vi "add data indicies controls.vi"(8 "error in":errorcluster, 9 "Channels to create":T1[](array[typedef]), 10 "runtime class path":path, 11 "Application in":refnum<vi>) -> (0 "error out":errorcluster)   [LabVIEW 2013, in "FixedChannelTBModuleDecideFeatures.lvclass"]
uses:
  FixedChannelTBModuleDecideFeatures.lvclass
  <vilib>/NI/Tag Bus Module Framework/channel/channel classification.ctl
  <vilib>/NI/Tag Bus Module Framework/channel/TBM channel.lvclass
  <vilib>/NI/Tag Bus/tag/Data Type.ctl
  <vilib>/NI/Tag Bus/tag/tag descriptor.lvclass
  channel configuration.ctl
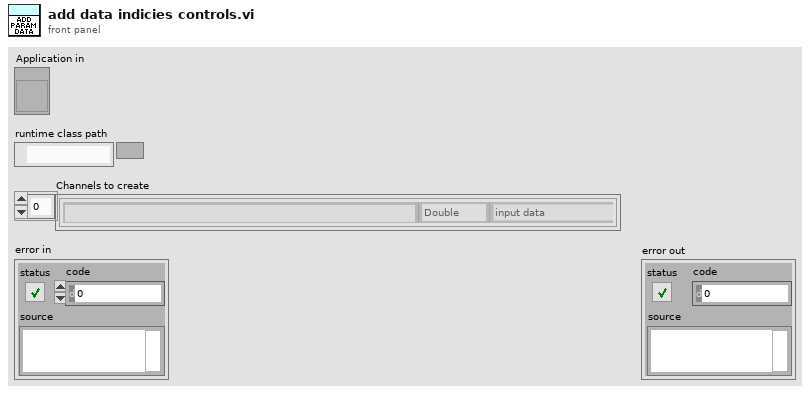
[diagram p1: front panel]
types:
  T1 = typedef "FixedChannelTBModuleDecideFeatures.lvclass/channel configuration.ctl" = cluster{"Name":string, "channel classification":T2, "data type":T3}
  T2 = typedef "TBM channel.lvclass/channel classification.ctl" = enum16{"input data", "output data", "processing parameter", "processing result"}
  T3 = typedef "tag bus.lvlib/tag descriptor.lvclass/Data Type.ctl" = enum16{"Double", "Single", "I64", "I32", "I16", "I8", "U64", "U32", "U16", "U8", "Boolean", "String", "Array of Double", "Array of Single", "Array of I64", "Array of I32", "Array of I16", "Array of I8", "Array of U64", "Array of U32", "Array of U16", "Array of U8", "Array of Boolean", "Array of String"}
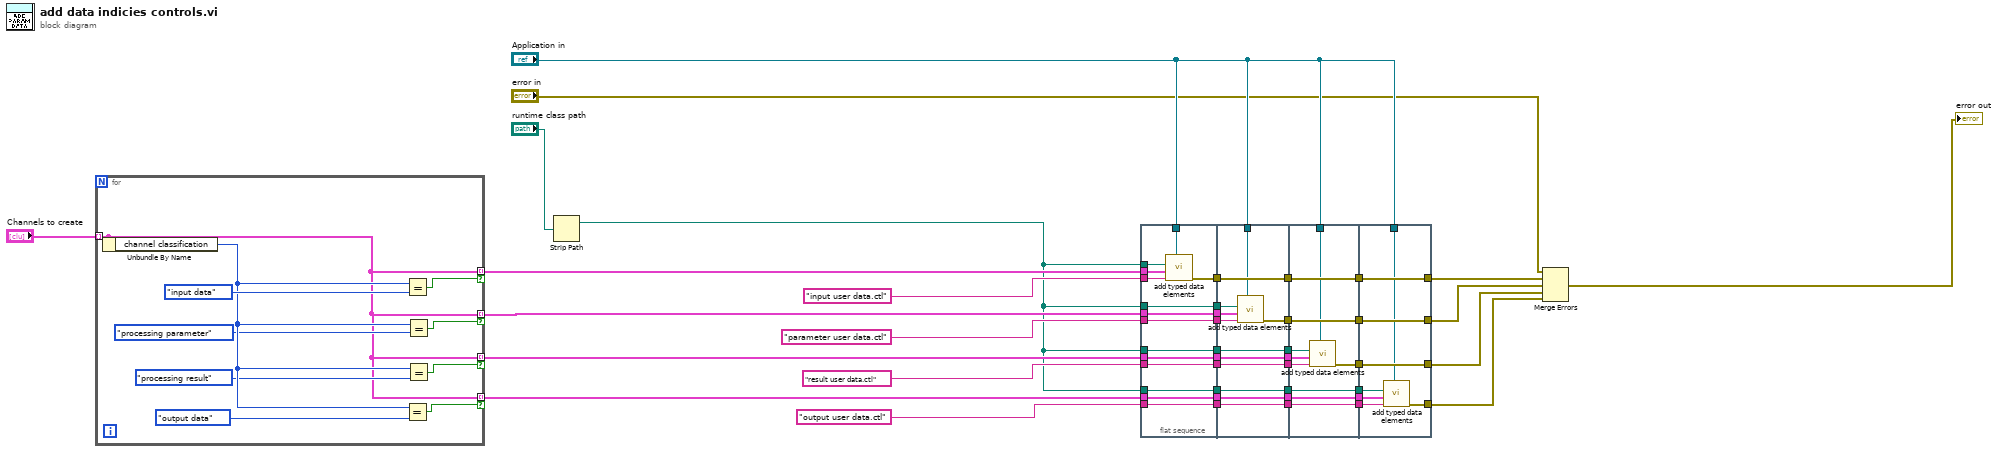
[diagram p0: block diagram]
diagram:
  n1 = for {
    tunnel: "Channels to create" -> [w43] mode=indexing
    tunnel: [w43] -> w39 mode=indexing if=w51
    tunnel: [w43] -> w36 mode=indexing if=w50
    tunnel: [w43] -> w28 mode=indexing if=w48
    tunnel: [w43] -> w20 mode=indexing if=w49
    n2 = Unbundle By Name(w43) -> ("channel classification"=w47:T2)
    n3 = Equal?(x=w47, y=channel_classification."output data" ("x")) -> (x = y?=w49:bool)
    n4 = Equal?(x=w47, y=channel_classification."input data" ("x")) -> (x = y?=w51:bool)
    n5 = Equal?(x=w47, y=channel_classification."processing parameter" ("x")) -> (x = y?=w50:bool)
    n6 = Equal?(x=w47, y=channel_classification."processing result" ("x")) -> (x = y?=w48:bool)
  }
  n7 = Strip Path(path="runtime class path") -> (stripped path=w21:path)  [unwired: 1 out]
  n8 = flat-sequence {
    tunnel: w39 -> [w53]
    tunnel: "input user data.ctl" ("name or relative path") -> [w66]
    tunnel: w21 -> [w65]
    tunnel: [w64] -> w37
    tunnel: w21 -> [w64]
    tunnel: w36 -> [w63]
    tunnel: [w63] -> w35
    tunnel: [w62] -> w34
    tunnel: "parameter user data.ctl" ("name or relative path") -> [w62]
    tunnel: [w61] -> w31
    tunnel: w21 -> [w61]
    tunnel: [w60] -> w29
    tunnel: w28 -> [w60]
    tunnel: "result user data.ctl" ("name or relative path") -> [w59]
    tunnel: [w59] -> w25
    tunnel: [w58] -> w22
    tunnel: w21 -> [w58]
    tunnel: w20 -> [w57]
    tunnel: [w57] -> w19
    tunnel: [w56] -> w14
    tunnel: "output user data.ctl" ("name or relative path") -> [w56]
    tunnel: [w55] -> w9
    tunnel: "Application in" -> [w54]
    tunnel: w37 -> [w78]
    tunnel: w35 -> [w67]
    tunnel: w34 -> [w77]
    tunnel: [w76] -> w32
    tunnel: w31 -> [w76]
    tunnel: [w75] -> w30
    tunnel: w29 -> [w75]
    tunnel: [w74] -> w26
    tunnel: w25 -> [w74]
    tunnel: [w73] -> w23
    tunnel: w22 -> [w73]
    tunnel: w19 -> [w72]
    tunnel: [w72] -> w18
    tunnel: [w71] -> w15
    tunnel: w14 -> [w71]
    tunnel: [w70] -> w10
    tunnel: w9 -> [w70]
    tunnel: [w69] -> w7
    tunnel: "Application in" -> [w68]
    tunnel: w32 -> [w88]
    tunnel: w30 -> [w79]
    tunnel: w26 -> [w87]
    tunnel: [w86] -> w24
    tunnel: w23 -> [w86]
    tunnel: w18 -> [w85]
    tunnel: [w85] -> w17
    tunnel: [w84] -> w16
    tunnel: w15 -> [w84]
    tunnel: [w83] -> w11
    tunnel: w10 -> [w83]
    tunnel: [w82] -> w8
    tunnel: w7 -> [w82]
    tunnel: [w81] -> w6
    tunnel: "Application in" -> [w80]
    tunnel: w24 -> [w96]
    tunnel: w17 -> [w89]
    tunnel: w16 -> [w95]
    tunnel: [w94] -> w12
    tunnel: w11 -> [w94]
    tunnel: [w93] -> w5
    tunnel: w8 -> [w93]
    tunnel: [w92] -> w4
    tunnel: w6 -> [w92]
    tunnel: [w91] -> w3
    tunnel: "Application in" -> [w90]
    frame #0 {
      n9 = call "add typed data elements.vi"("Application in"=w54, "Typedef relative path"=w66, "Channels to create"=w53, "cfg class base path"=w65) -> ("error out"=w55:errorcluster)  [unwired: 7 in]
    }
    frame #1 {
      n10 = call "add typed data elements.vi"("Application in"=w68, "Typedef relative path"=w77, "Channels to create"=w67, "cfg class base path"=w78) -> ("error out"=w69:errorcluster)  [unwired: 7 in]
    }
    frame #2 {
      n11 = call "add typed data elements.vi"("Application in"=w80, "Typedef relative path"=w87, "Channels to create"=w79, "cfg class base path"=w88) -> ("error out"=w81:errorcluster)  [unwired: 7 in]
    }
    frame #3 {
      n12 = call "add typed data elements.vi"("Application in"=w90, "Typedef relative path"=w95, "Channels to create"=w89, "cfg class base path"=w96) -> ("error out"=w91:errorcluster)  [unwired: 7 in]
    }
  }
  n13 = Merge Errors("error in", w12, w5, w4, w3) -> (→"error out":errorcluster)
